vi "GUI_laptop v11d.vi"() -> ()   [LabVIEW 2019]
uses:
  <vilib>/Math Plots/3D Math Plots/3D Scatter/3D Scatter XCtrl/3D Scatter.xctl
  <vilib>/Platform/TimedLoop/XDataNode/timing_clust.ctl
  <vilib>/Platform/TimedLoop/XDataNode/nitl_modes.ctl
  <vilib>/Platform/TimedLoop/XDataNode/wakeup.ctl
  <vilib>/Analysis/_algsub.llb/Real Vector Norm.vi
  <vilib>/Instr/_visa.llb/VISA Configure Serial Port (Instr).vi
  <vilib>/Utility/file.llb/Write Delimited Spreadsheet (DBL).vi
  <vilib>/Math Plots/3D Math Plots/3D Scatter/3D Scatter Datatype/Public/Plot Helper (Vector).vi
  <vilib>/platform/TimedLoop/XDataNode/XDataNode.xnode
  <vilib>/Platform/TimedLoop/XDataNode/XDNodeRunTimeDep.lvlib
  <vilib>/Analysis/NI_AALPro.lvlib
  <vilib>/Math Plots/3D Math Plots/3D Scatter/3D Scatter Datatype/3D Scatter Datatype.lvclass
panel:
  in  "Motion Scale L4":dbl=2.0
  out "spreadsheet string":string
  in  "Save Path 2":path=path "C:/Users/jimmy/Documents/GitHub/Arduino-LabVIEW/zhantao/read_data_delt.csv"
  out "Numeric":i32
  out "send values":dbl[](array[numeric])
  out "Robot Feedback (xyz)":dbl[](array[numeric])
  in  "UDP Send":bool
  in  "UDP Recv":bool
  in  "L5 bound":dbl=1000.0
  in  "L4 bound (deg)":dbl=1000.0
  in  "L3 bound (mm)":dbl=1000.0
  in  "L2 bound (deg)":dbl=1000.0
  in  "L1 bound (deg)":dbl=1000.0
  in  "Joystick Type":dbl(ring) items=["Rigid Joystick", "Free Joystick"]
  out "Finished Late? [i-1]":bool
  in  "Epsilon":dbl=0.2
  out "3D Scatter":refnum<class "3D Plot Datatype.lvclass">[](xcontrol)
  out "Random Point":dbl[](array[numeric])
  out "Virtual Cursor":dbl[](array[numeric])
  out "Iteration Duration":i64
  in  "Num of Points":i32=10
  in  "z bound":dbl=2.0
  in  "y bound":dbl=5.0
  in  "x bound":dbl=5.0
  in  "Stop":bool
  in  "Round Decimals":dbl=2.0 format="%#_15g"
  in  "Save  Data":bool
  in  "Save Path":path=path "C:/Users/jimmy/Documents/GitHub/Arduino-LabVIEW/zhantao/read_data_abs.csv"
  in  "x speed":dbl=0.5
  in  "z speed":dbl=0.5
  in  "y speed":dbl=0.5
  out "error out":errorcluster
  in  "baud rate":u32=115200
  in  "VISA resource name":refnum<visa-resource-name>
  # "TODO: fix the bounds; currently bounds are arbitrary"
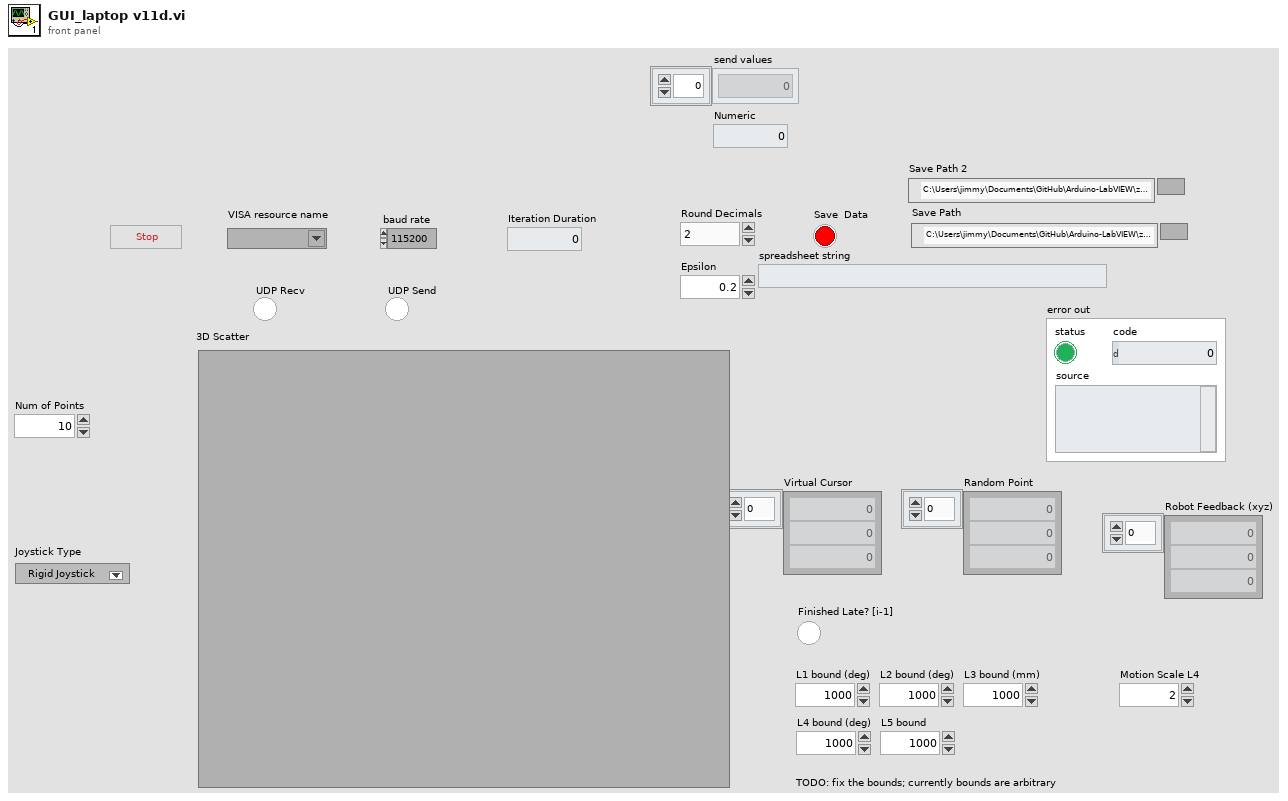
[diagram p1: front panel]
types:
  T1 = typedef "XDNodeRunTimeDep.lvlib/timing_clust.ctl" = cluster{"Expected End [f-1]":u64, "Actual End [f-1]":u64, "Finished Late? [f-1]":bool, "Expected End [i-1]":u64, "Actual End [i-1]":u64, "Finished Late? [i-1]":bool, "Expected Start [i]":u64, "Actual Start [i]":u64, "Expected Start [f]":u64, "Actual Start [f]":u64, "Source Name":string, "Structure Name":string, "Period":i64, "Deadline":i64, "Offset":i64, "Start":i64, "Priority":i32, "Timeout":i32, "Mode":T2, "Wakeup Reason":T3, "Error":errorcluster, "Source Type":string, "Secondary Source Type":string, "Global End Time":u64, "Global Start Time":u64, "Frame Duration":u64, "Iteration Duration":u64, "Assigned CPU":i32, "I/O Scan Engine Mode":u32}
  T2 = typedef "XDNodeRunTimeDep.lvlib/nitl_modes.ctl" = enum32{"No Change", "Process missed periods, maintain original phase", "Discard missed periods, maintain original phase", "Process missed periods, ignore original phase", "Discard missed periods, ignore original phase"}
  T3 = typedef "XDNodeRunTimeDep.lvlib/wakeup.ctl" = enum32{"Normal", "Aborted", "Asynchronous wakeup", "Timing source error", "Timed loop error", "Timeout"}
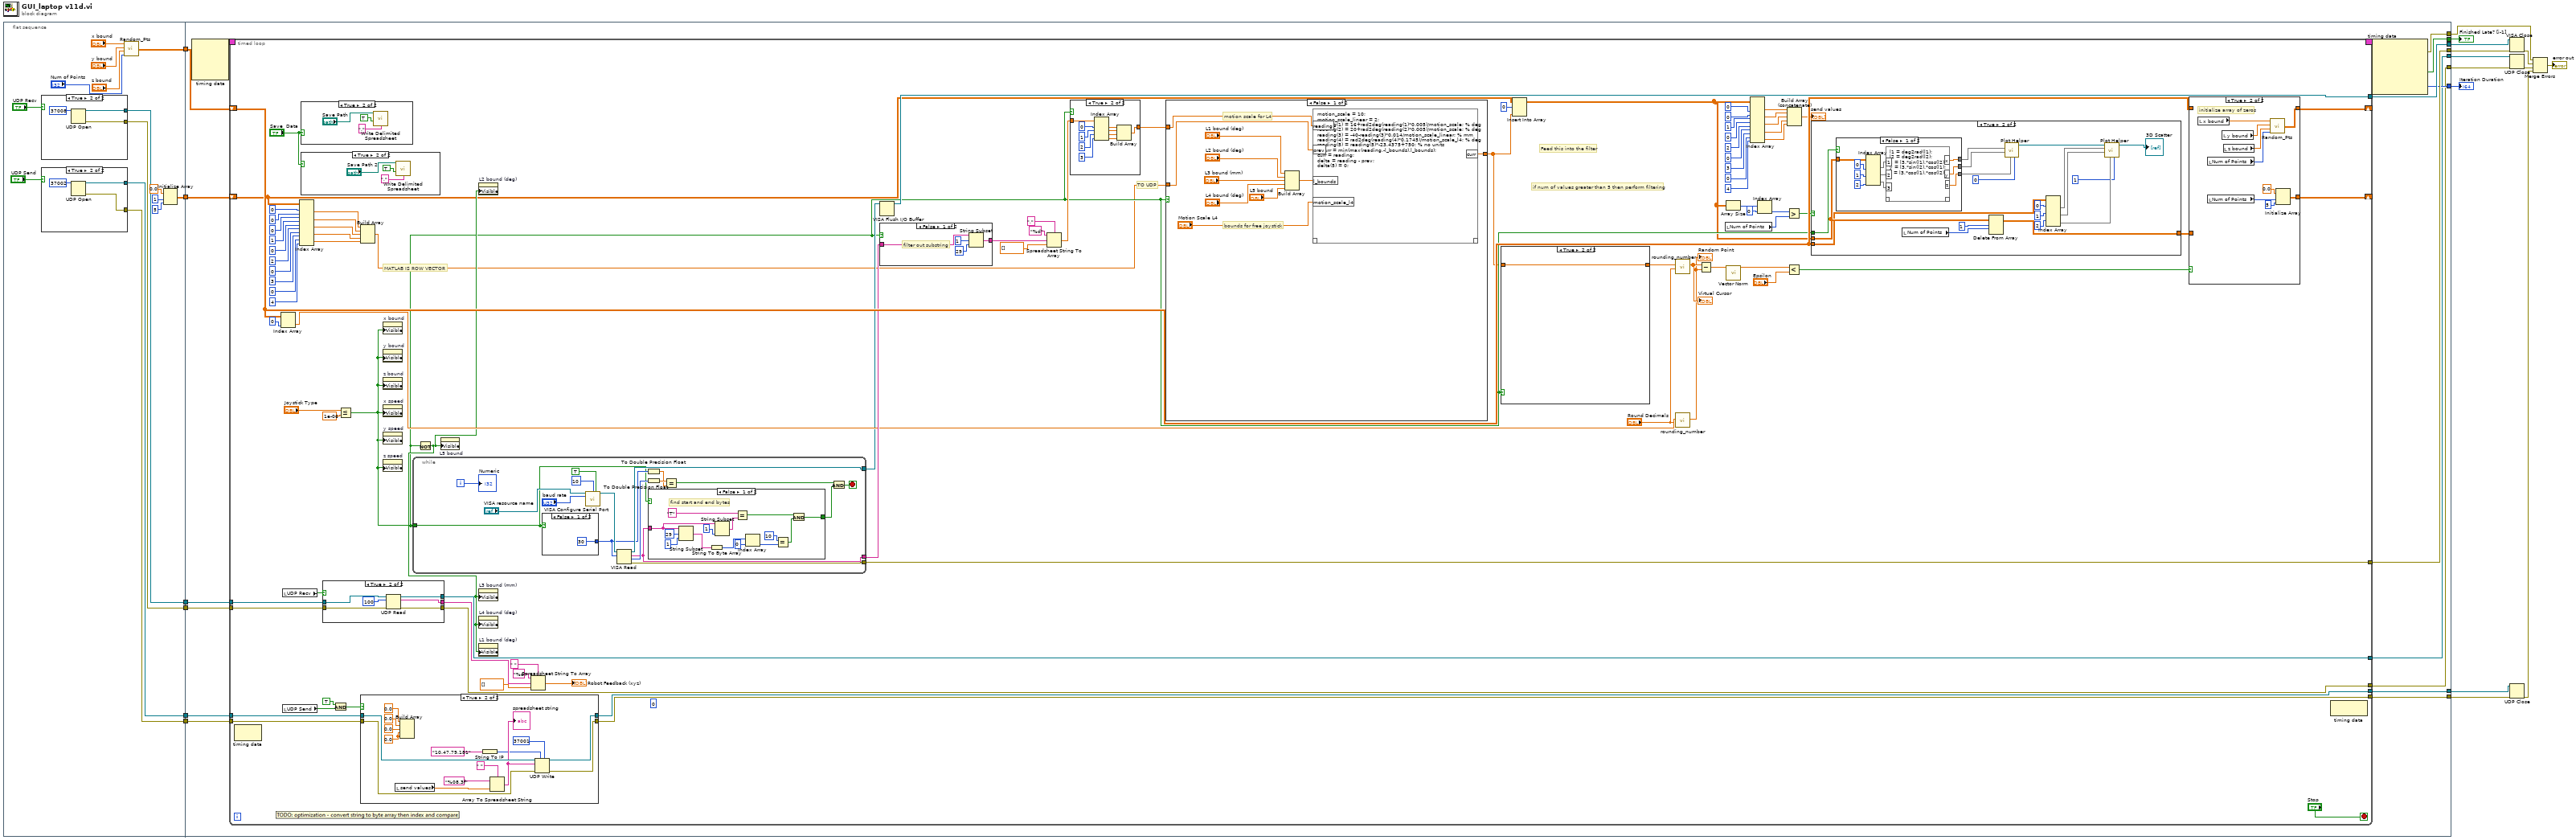
[diagram p0: block diagram]
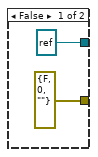
[diagram p2: hidden frame]
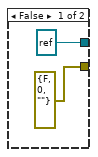
[diagram p3: hidden frame]
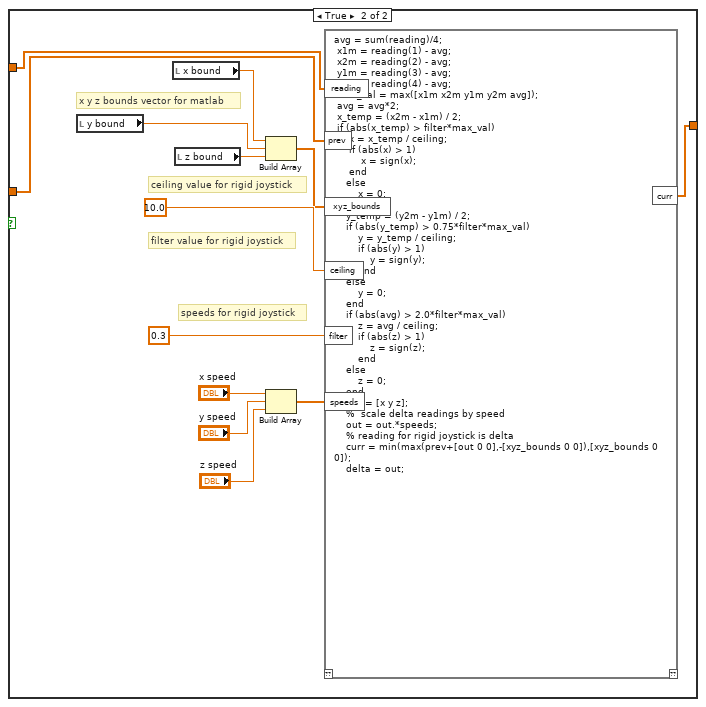
[diagram p4: hidden frame]
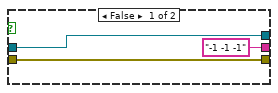
[diagram p7: hidden frame]
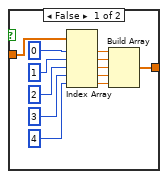
[diagram p11: hidden frame]
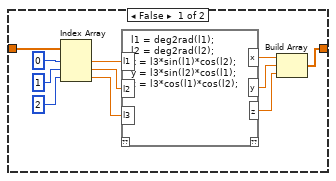
[diagram p12: hidden frame]
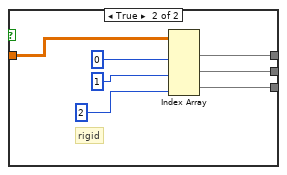
[diagram p14: hidden frame]
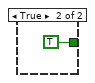
[diagram p15: hidden frame]
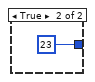
[diagram p16: hidden frame]
diagram:
  n1 = flat-sequence {
    tunnel: [w26] -> w15
    tunnel: [w30] -> w14
    tunnel: [w25] -> w13
    tunnel: [w24] -> w12
    tunnel: [w21] -> w11
    tunnel: [w20] -> w10
    tunnel: [w59] -> w19
    tunnel: [w58] -> w18
    tunnel: [w56] -> w9
    tunnel: [w54] -> w17
    tunnel: [w53] -> w16
    tunnel: w15 -> [w57]
    tunnel: w14 -> [w55]
    tunnel: w13 -> [w52]
    tunnel: w12 -> [w51]
    tunnel: w11 -> [w50]
    tunnel: w10 -> [w49]
    tunnel: [w48] -> w3
    tunnel: [w47] -> w8
    tunnel: [w46] -> w2
    tunnel: [w45] -> w1
    frame #0 {
      n2 = case shown="True" "UDP Recv" {
        tunnel: [refnum<k16> refnum ("port") w43] -> w24
        tunnel: [errorcluster {"status"=FALSE, "code"=0, "source"=""} ("error out") w42] -> w21
        frame False {
        }
        frame True {
          n3 = UDP Open(11:u16 37008 ("port")) -> (port=w43:refnum<k16>, 0:w42:errorcluster)  [unwired: 4 in, 1 out]
        }
      }
      n4 = case shown="True" "UDP Send" {
        tunnel: [refnum<k16> refnum ("port") w38] -> w25
        tunnel: [errorcluster {"status"=FALSE, "code"=0, "source"=""} ("error out") w37] -> w20
        frame False {
        }
        frame True {
          n5 = UDP Open(11:u16 37002 ("port")) -> (port=w38:refnum<k16>, 0:w37:errorcluster)  [unwired: 4 in, 1 out]
        }
      }
      n6 = call "Random_Pts.vi"("Num of Points"="Num of Points", "z bound"="z bound", "y bound"="y bound", "x bound"="x bound") -> ("appended array"=w30:dbl[][])
      n7 = Initialize Array(0.0 ("element"), 1 ("dimension size"), 5 ("dimension size")) -> (w26:dbl[][])
    }
    frame #1 {
      n8 = node-c288() -> (w61:T1)  [unwired: 4 in]
      n9 = timed-loop {
        tunnel: [w87] -> w59
        tunnel: [w147] -> w58
        shift-right: [w146] -> _
        shift-left: w57 -> [w64]
        timing: w61 -> [_]
        timing-out: [_] -> w60
        shift-right: [w142] -> _
        shift-left: w55 -> [w143]
        tunnel: w52 -> [w105]
        tunnel: w51 -> [w104]
        tunnel: w50 -> [w102]
        tunnel: w49 -> [w101]
        tunnel: [w100] -> w48
        tunnel: [w99] -> w47
        tunnel: [w98] -> w46
        tunnel: [w97] -> w45
        stop <- "Stop" stop-if-true
        (unwired) 0 ("disabled index (row)")
        # "if num of values greater than 5 then perform filtering"
        # "Feed this into the filter"
        # "TO UDP"
        # "MATLAB IS ROW VECTOR"
        n10 = node-c288() -> ()  [unwired: 1 in, 1 out]
        n11 = Index Array(array=w143, index (col)=0 ("index (row)")) -> (element=w114:dbl[])  [unwired: 1 in]
        n12 = local read "UDP Recv"() -> (w103:bool)
        n13 = local read "UDP Send"() -> (w91:bool)
        n14 = Index Array(array=w64, index (row) #1=0 ("disabled index (row)"), index (col) #1=0 ("disabled index (col)"), index (row) #2=0 ("disabled index (row)"), index (col) #2=1 ("disabled index (col)"), index (row) #3=0 ("disabled index (row)"), index (col) #3=2 ("disabled index (col)"), index (row) #4=0 ("disabled index (row)"), index (col) #4=3 ("disabled index (col)"), index (row) #5=0 ("disabled index (row)"), index (col) #5=4 ("disabled index (col)")) -> (element #1=w128:dbl, element #2=w127:dbl, element #3=w126:dbl, element #4=w119:dbl, element #5=w118:dbl)
        n15 = case shown="True" "Save  Data" {
          frame False {
          }
          frame True {
            n16 = call-poly <vilib>:"Write Delimited Spreadsheet.vi"("file path (dialog if empty)"="Save Path", "append to file? (new file:F)"=TRUE, "delimiter (\\t)"="," ("delimiter (\\t)")) -> ()  [unwired: 11 in, 2 out]
          }
        }
        n17 = case shown="True" "Save  Data" {
          frame False {
          }
          frame True {
            n18 = call-poly <vilib>:"Write Delimited Spreadsheet.vi"("file path (dialog if empty)"="Save Path 2", "append to file? (new file:F)"=TRUE, "delimiter (\\t)"="," ("delimiter (\\t)")) -> ()  [unwired: 11 in, 2 out]
          }
        }
        n19 = case shown="True" w103 {
          tunnel: w104 -> [w193 w200]
          tunnel: w102 -> [w194 w199]
          tunnel: [w194 w198] -> w100
          tunnel: [w193 w197] -> w98
          tunnel: ["-1 -1 -1" w195] -> w93
          frame False {
          }
          frame True {
            n20 = UDP Read(connection ID=w200, max size (548)=100, 8:w199) -> (data out=w195:string, error out=w198:errorcluster, 3:w197:refnum<k16>)  [unwired: 1 in, 2 out]
          }
        }
        n21 = And(x=TRUE, y=w91) -> (x .and. y?=w90:bool)
        n22 = Less Or Equal?(x="Joystick Type", y=1e-06) -> (x <= y?=w84:bool)
        n23 = Build Array(w128, w127, w126, w119, w118) -> (w83:dbl[])
        n24 = case shown="True" w90 {
          tunnel: w105 -> [w175 w191]
          tunnel: w101 -> [w176 w187]
          tunnel: [w176 w183] -> w99
          tunnel: [w175 w182] -> w97
          frame False {
          }
          frame True {
            w181 = 0.0 ("element")
            n25 = local read "send values"() -> (w177:dbl[])
            n26 = Build Array(0.0 ("element"), 0.0 ("element"), 0.0 ("element"), w181, w181) -> ()  [unwired: 1 out]
            n27 = String To IP(1:"10.47.79.181" ("name")) -> (0:w185:u32)
            n28 = Array To Spreadsheet String(delimiter (Tab)=" ", array=w177, 3:"%08.3f" ("format string")) -> (spreadsheet string=w188:string)
            "spreadsheet string" <- w188
            n29 = UDP Write(address=w185, port or service name=u16 37001, connection ID=w191, data in=w188, 8:w187) -> (error out=w183:errorcluster, 3:w182:refnum<k16>)  [unwired: 1 in]
          }
        }
        n30 = property on="x bound" class="DigNum (strict)"("Visible"=w84) -> ()  [unwired: 2 in, 2 out]
        n31 = property on="y bound" class="DigNum (strict)"("Visible"=w84) -> ()  [unwired: 2 in, 2 out]
        n32 = property on="z bound" class="DigNum (strict)"("Visible"=w84) -> ()  [unwired: 2 in, 2 out]
        n33 = property on="x speed" class="DigNum (strict)"("Visible"=w84) -> ()  [unwired: 2 in, 2 out]
        n34 = property on="y speed" class="DigNum (strict)"("Visible"=w84) -> ()  [unwired: 2 in, 2 out]
        n35 = property on="z speed" class="DigNum (strict)"("Visible"=w84) -> ()  [unwired: 2 in, 2 out]
        n36 = while {
          tunnel: [w292] -> w116
          tunnel: [w305] -> w147
          tunnel: [w299] -> w88
          tunnel: w84 -> [w293]
          i -> [w291]
          stop <- w295 stop-if-true
          n37 = case shown="False" w293 {
            tunnel: [30 u32 23 ("byte count")] -> w298
            frame False {
            }
            frame True {
            }
          }
          n38 = call-poly "VISA Configure Serial Port"("VISA resource name"="VISA resource name", "termination char\n(0xA = '\\n' = LF)"=u8 10 ("termination char\n(0xA = '\\n' = LF)"), "Enable Termination\nChar (T)"=TRUE ("Enable Termination\nChar (T)"), "baud rate (9600)"="baud rate") -> ("VISA resource name out"=w300:refnum<visa-resource-name>)  [unwired: 10 in, 1 out]
          n39 = VISA Read(VISA resource name=w300, byte count=w298) -> (VISA resource name out=w299:refnum<visa-resource-name>, read buffer=w292:string, return count=w307:u32, error out=w305:errorcluster)  [unwired: 1 in]
          n40 = To Double Precision Float(number=w298) -> (double precision float=w297:dbl)
          n41 = To Double Precision Float(number=w307) -> (double precision float=w306:dbl)
          n42 = case shown="False" w293 {
            tunnel: [w314 TRUE] -> w294
            tunnel: w292 -> [w317 _]
            frame False {
              # "find start and end bytes"
              n43 = String Subset(string=w317, offset (0)=29, length (rest)=1) -> (substring=w312:string)
              n44 = String To Byte Array(string=w312) -> (unsigned byte array=w311:u8[])
              n45 = String Subset(string=w317, length (rest)=1) -> (substring=w320:string)  [unwired: 1 in]
              n46 = Equal?(x="T", y=w320) -> (x = y?=w316:bool)
              n47 = Index Array(array=w311, index=0) -> (element=w309:u8)
              n48 = Equal?(x=10, y=w309) -> (x = y?=w315:bool)
              n49 = And(x=w316, y=w315) -> (x .and. y?=w314:bool)
            }
            frame True {
            }
          }
          n50 = Equal?(x=w306, y=w297) -> (x = y?=w296:bool)
          n51 = And(x=w296, y=w294) -> (x .and. y?=w295:bool)
          "Numeric" <- w291
        }
        n52 = Not(x=w84) -> (.not. x?=w89:bool)
        n53 = property on="L5 bound" class="DigNum (strict)"("Visible"=w89) -> ()  [unwired: 2 in, 2 out]
        n54 = property on="L2 bound (deg)" class="DigNum (strict)"("Visible"=w89) -> ()  [unwired: 2 in, 2 out]
        n55 = property on="L3 bound (mm)" class="DigNum (strict)"("Visible"=w89) -> ()  [unwired: 2 in, 2 out]
        n56 = property on="L4 bound (deg)" class="DigNum (strict)"("Visible"=w89) -> ()  [unwired: 2 in, 2 out]
        n57 = property on="L1 bound (deg)" class="DigNum (strict)"("Visible"=w89) -> ()  [unwired: 2 in, 2 out]
        n58 = Spreadsheet String To Array(delimiter (Tab)=" ", format string="%d", spreadsheet string=w93, array type (2D Dbl)=dbl[] []) -> (array=→"Robot Feedback (xyz)":dbl[])
        n59 = VISA Flush I/O Buffer(VISA resource name=w88) -> (VISA resource name out=w87:refnum<visa-resource-name>)  [unwired: 2 in, 1 out]
        n60 = case shown="False" w84 {
          tunnel: w116 -> [w218 w219]
          tunnel: [w215 w219] -> w115
          frame False {
            # "filter out substring"
            n61 = String Subset(string=w218, offset (0)=1, length (rest)=29) -> (substring=w215:string)
          }
          frame True {
          }
        }
        n62 = Spreadsheet String To Array(delimiter (Tab)=",", format string="%d", spreadsheet string=w115, array type (2D Dbl)=dbl[] []) -> (array=w117:dbl[])
        n63 = case shown="True" w84 {
          tunnel: w117 -> [w220 w235]
          tunnel: [w225 w234] -> w82
          frame False {
            n64 = Index Array(array=w220, index #1=0 ("Plot ID"), index #2=1 ("Plot ID"), index #3=2 ("Plot ID"), index #4=3 ("Plot ID"), index #5=4 ("Plot ID")) -> (element #1=w228:dbl, element #2=w227:dbl, element #3=w226:dbl, element #4=w222:dbl, element #5=w221:dbl)
            n65 = Build Array(w228, w227, w226, w222, w221) -> (w225:dbl[])
          }
          frame True {
            n66 = Index Array(array=w235, index #1=0 ("Plot ID"), index #2=1 ("Plot ID"), index #3=2 ("Plot ID"), index #4=3 ("index")) -> (element #1=w238:dbl, element #2=w237:dbl, element #3=w236:dbl, element #4=w232:dbl)
            n67 = Build Array(w238, w237, w236, w232) -> (w234:dbl[])
          }
        }
        n68 = case shown="False" w84 {
          tunnel: w83 -> [w150 w161]
          tunnel: w82 -> [w151 w160]
          tunnel: [w149 w159] -> w62
          frame False {
            # "bounds for free joystick"
            # "motion scale for L4"
            n69 = Build Array("L1 bound (deg)", "L2 bound (deg)", "L3 bound (mm)", "L4 bound (deg)", "L5 bound") -> (w152:dbl[])
            n70 = script code="motion_scale = 10;\nmotion_scale_linear = 2;\nreading(1) = 16+rad2deg(reading(1)*0.005)/motion_scale; % deg\nreading(2) = 20+rad2deg(reading(2)*0.005)/motion_scale; % deg\nreading(3) = -40-reading(3)*0.014/motion_scale_linear; % mm\nreading(4) = rad2deg(reading(4)*0.1745)/motion_scale_l4; % deg\nreading(5) = reading(5)*-23.4375+750; % no units\n%curr = min(max(reading,-l_bounds),l_bounds);\ncurr = reading;\ndelta = reading - prev;\ndelta(5) = 0;"("l_bounds"=w152, "motion_scale_l4"="Motion Scale L4", "reading"=w151, "prev"=w150) -> ("curr"=w149:dbl[])  [unwired: 1 in, 1 out]
          }
          frame True {
            # "ceiling value for rigid joystick"
            # "filter value for rigid joystick"
            # "speeds for rigid joystick"
            # "x y z bounds vector for matlab"
            n71 = local read "y bound"() -> (w170:dbl)
            n72 = local read "x bound"() -> (w169:dbl)
            n73 = local read "z bound"() -> (w171:dbl)
            n74 = Build Array(w169, w170, w171) -> (w162:dbl[])
            n75 = Build Array("x speed", "y speed", "z speed") -> (w165:dbl[])
            n76 = script code="avg = sum(reading)/4;\n x1m = reading(1) - avg;\n x2m = reading(2) - avg;\n y1m = reading(3) - avg;\n y2m = reading(4) - avg;\n max_val = max([x1m x2m y1m y2m avg]);\n avg = avg*2;\n x_temp = (x2m - x1m) / 2;\n if (abs(x_temp) > filter*max_val)\n     x = x_temp / ceiling;\n     if (abs(x) > 1)\n         x = sign(x);\n     end\n    else\n        x = 0;\n    end\n    y_temp = (y2m - y1m) / 2;\n    if (abs(y_temp) > 0.75*filter*max_val)\n        y = y_temp / ceiling;\n        if (abs(y) > 1)\n            y = sign(y);\n        end\n    else\n        y = 0;\n    end\n    if (abs(avg) > 2.0*filter*max_val)\n        z = avg / ceiling;\n        if (abs(z) > 1)\n            z = sign(z);\n        end\n    else\n        z = 0;\n    end\n    out = [x y z];\n    %  scale delta readings by speed\n    out = out.*speeds;\n    % reading for rigid joystick is delta\n    curr = min(max(prev+[out 0 0],-[xyz_bounds 0 0]),[xyz_bounds 0 0]);\n    delta = out;"("xyz_bounds"=w162, "ceiling"=10.0 ("Real"), "filter"=0.3 ("Real"), "speeds"=w165, "reading"=w160, "prev"=w161) -> ("curr"=w159:dbl[])  [unwired: 1 in, 1 out]
          }
        }
        n77 = case shown="True" w84 {
          tunnel: [w246 w253] -> w144
          tunnel: w62 -> [w245 w253]
          frame False {
            n78 = Index Array(array=w245, index #1=0 ("Plot ID"), index #2=1 ("Plot ID"), index #3=2 ("Plot ID")) -> (element #1=w244:dbl, element #2=w243:dbl, element #3=w242:dbl)
            n79 = script code="l1 = deg2rad(l1);\nl2 = deg2rad(l2);\nx = l3*sin(l1)*cos(l2);\ny = l3*sin(l2)*cos(l1);\nz = l3*cos(l1)*cos(l2);"("l1"=w244, "l2"=w243, "l3"=w242) -> ("x"=w249:dbl, "y"=w248:dbl, "z"=w247:dbl)  [unwired: 1 in, 1 out]
            n80 = Build Array(w249, w248, w247) -> (w246:dbl[])
          }
          frame True {
          }
        }
        n81 = Insert Into Array(array=w64, index (row)=0, new element=w62) -> (w63:dbl[][])  [unwired: 1 in]
        n82 = call "rounding_number.vi"("power of ten"="Round Decimals", "Array"=w144) -> ("rounded"=w112:dbl[])  [unwired: 9 in]
        "Virtual Cursor" <- w112
        n83 = call "rounding_number.vi"("power of ten"="Round Decimals", "Array"=w114) -> ("rounded"=w111:dbl[])  [unwired: 9 in]
        "Random Point" <- w111
        n84 = Subtract(x=w112, y=w111) -> (x-y=w110:dbl[])
        n85 = local read "Num of Points"() -> (w130:i32)
        n86 = Array Size(array=w63) -> (size(s)=w81:i32[])
        n87 = call-poly <vilib>:"Vector Norm.vi"("Input Vector"=w110) -> ("norm"=w109:dbl)  [unwired: 9 in, 1 out]
        n88 = Index Array(array=w63, index (col) #1=0 ("disabled index (col)"), index (row) #2=0 ("disabled index (row)"), index (col) #2=1 ("disabled index (col)"), index (row) #3=0 ("disabled index (row)"), index (col) #3=2 ("disabled index (col)"), index (row) #4=0 ("disabled index (row)"), index (col) #4=3 ("disabled index (col)"), index (row) #5=0 ("disabled index (row)"), index (col) #5=4 ("disabled index (col)")) -> (element #1=w75:dbl[], element #2=w74:dbl, element #3=w73:dbl, element #4=w68:dbl, element #5=w67:dbl)  [unwired: 1 in]
        n89 = Index Array(array=w81, index=0) -> (element=w131:i32)
        n90 = Greater?(x=w131, y=w130) -> (0:w129:bool)
        n91 = Less?(x=w109, y="Epsilon") -> (x < y?=w107:bool)
        n92 = Build Array (concatenate)(w75, w74, w73, w68, w67) -> (→"send values":dbl[])
        n93 = case shown="True" w129 {
          tunnel: w63 -> [w254 w272]
          tunnel: [w254 w271] -> w145
          tunnel: w143 -> [_ w270]
          tunnel: w84 -> [_ w255]
          frame False {
          }
          frame True {
            n94 = case shown="False" w255 {
              tunnel: w272 -> [w283 w287]
              tunnel: [w274 w286] -> w261
              tunnel: [w275 w285] -> w260
              tunnel: [w276 w284] -> w259
              frame False {
                n95 = Index Array(array=w283, index (col) #1=0 ("Plot ID"), index (col) #2=1 ("Plot ID"), index (col) #3=2 ("Plot ID")) -> (element #1=w279:dbl[], element #2=w278:dbl[], element #3=w277:dbl[])  [unwired: 3 in]
                n96 = script code="l1 = deg2rad(l1);\nl2 = deg2rad(l2);\nx = l3.*sin(l1).*cos(l2);\ny = l3.*sin(l2).*cos(l1);\nz = l3.*cos(l1).*cos(l2);"("l1"=w279, "l2"=w278, "l3"=w277) -> ("x"=w274:dbl[], "y"=w275:dbl[], "z"=w276:dbl[])  [unwired: 1 in, 1 out]
              }
              frame True {
                # "rigid"
                n97 = Index Array(array=w287, index (col) #1=0 ("disabled index (col)"), index (col) #2=1 ("index (col)"), index (col) #3=2 ("index (col)")) -> (element #1=w286:dbl[], element #2=w285:dbl[], element #3=w284:dbl[])  [unwired: 3 in]
              }
            }
            n98 = local read "Num of Points"() -> (w269:i32)
            n99 = Delete From Array(array=w272, length=1, index (row)=w269) -> (array with subset deleted=w271:dbl[][])  [unwired: 1 in, 1 out]
            n100 = call-poly <vilib>:"Plot Helper.vi"("Plot ID"=0, "z vector"=w259, "y vector"=w260, "x vector"=w261) -> ("3D Plot lvclass Array out"=w263:refnum<class "3D Plot Datatype.lvclass">[])  [unwired: 2 in, 5 out]
            n101 = Index Array(array=w270, index (row) #1=0 ("index (row)"), index (row) #2=1 ("index (row)"), index (row) #3=2 ("index (row)")) -> (element #1=w267:dbl[], element #2=w266:dbl[], element #3=w265:dbl[])  [unwired: 3 in]
            n102 = call-poly <vilib>:"Plot Helper.vi"("Plot ID"=1, "z vector"=w265, "y vector"=w266, "x vector"=w267, "3D Plot lvclass Array in"=w263) -> ("3D Plot lvclass Array out"=→"3D Scatter":refnum<class "3D Plot Datatype.lvclass">[])  [unwired: 1 in, 5 out]
          }
        }
        n103 = case shown="True" w107 {
          tunnel: w143 -> [w205 _]
          tunnel: [w205 w210] -> w142
          tunnel: w145 -> [w204 _]
          tunnel: [w204 w206] -> w146
          frame False {
          }
          frame True {
            # "initialize array of zeros"
            n104 = local read "x bound"() -> (w214:dbl)
            n105 = local read "Num of Points"() -> (w211:i32)
            n106 = local read "Num of Points"() -> (w208:i32)
            n107 = local read "y bound"() -> (w213:dbl)
            n108 = local read "z bound"() -> (w212:dbl)
            n109 = call "Random_Pts.vi"("Num of Points"=w211, "z bound"=w212, "y bound"=w213, "x bound"=w214) -> ("appended array"=w210:dbl[][])
            n110 = Initialize Array(0.0 ("element"), w208, 5 ("dimension size")) -> (w206:dbl[][])
          }
        }
        n111 = node-c288() -> ()  [unwired: 1 in, 1 out]
      }
      n112 = node-c288(w60) -> (w56:errorcluster, w53:bool, w54:i64)  [unwired: 3 out]
    }
  }
  n113 = VISA Close(VISA resource name=w19, error in (no error)=w18) -> (error out=w7:errorcluster)
  n114 = UDP Close(connection ID=w2, 8:w3) -> (error out=w6:errorcluster)  [unwired: 1 out]
  n115 = UDP Close(connection ID=w1, 8:w8) -> (error out=w5:errorcluster)  [unwired: 1 out]
  n116 = Merge Errors(w9, w7, w6, w5) -> (→"error out":errorcluster)
  "Iteration Duration" <- w17
  "Finished Late? [i-1]" <- w16
